vi "Test Copy To Raw Memory ARGB.vi"(8 "error in (no error)":errorcluster, 11 "Test Case In":refnum<class "01_Image.lvclass">) -> (0 "error out":errorcluster, 3 "Test Case Out":refnum<class "01_Image.lvclass">)   [LabVIEW 2020, in "test.lvlib" / "01_Image.lvclass"]
uses:
  01_Image.lvclass
  C:/Program Files (x86)/National Instruments/LabVIEW 2026/vi.lib/Astemes/LUnit/Test Case.lvclass
  common/Image Size (Integer).ctl
  image/Raw Memory Information.ctl
  image/Raw Memory Information Dimension.ctl
  <vilib>/Astemes/LUnit/Test Case.lvclass/Test Case.ctl
  4993e8ee-a06a-463a-9684-69129f64d5ce.vi
  image/New Image.vi
  image/New Image (ARGB Preallocated).vi
  image/Copy Array to Image.vi
  image/Copy Array to Image (ARGB).vi
  image/Copy Image to Memory Address (ARGB).vi/01eda17f-9221-4e43-bf47-cf9d986167a3.vi
  <vilib>/Astemes/LUnit/Core/LUnit Test Case/Private/Append Pass Result.vi
  <vilib>/Astemes/LUnit/Core/LUnit Test Case/Private/Append Fail Result.vi
  4993e8ee-a06a-463a-9684-69129f64d5ce.vi/9c5d11cd-9439-4240-a1ee-d9baace9c924.vi
  image/New Image (ARGB Preallocated).vi/3321fa97-f432-4e1e-8db9-a0df79aed21b.vi
  image/ARGB Colour to U32 Pixel Value.vi
  <vilib>/Astemes/LUnit/Core/LUnit Test Case/Private/Run In UI.vi
  <vilib>/Utility/error.llb/Clear Errors.vi
  <vilib>/Utility/error.llb/Error Cluster From Error Code.vi
  <vilib>/picture/pixmap.llb/Flatten Pixmap.vi
  image/image.lvlib
  common/common.lvlib
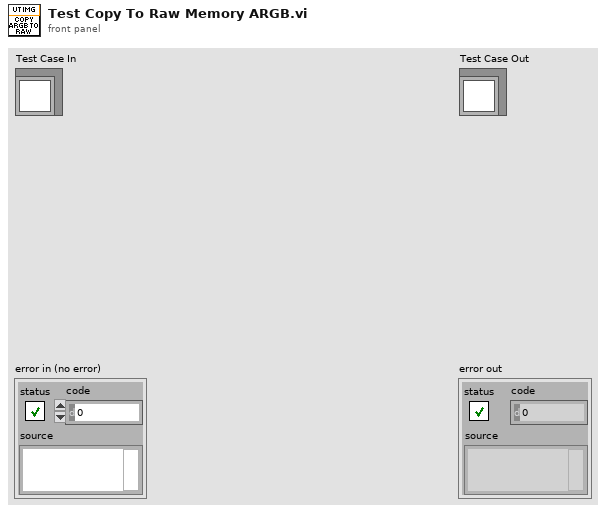
[diagram p1: front panel]
types:
  T1 = typedef "common.lvlib/Image Size (Integer).ctl" = cluster{"Width":u16, "Height":u16}
  T2 = typedef "image.lvlib/ARGB Image.ctl" = refnum<data-value>
  T3 = typedef "image.lvlib/Raw Memory Information.ctl" = cluster{"Memory Address":u64, "Dimension 0":T4, "Dimension 1":T4}
  T4 = typedef "image.lvlib/Raw Memory Information Dimension.ctl" = cluster{"Size":u16, "Stride":i32}
  T5 = cluster{"pointer":u64, "size_0":u32, "stride_0":i32, "size_1":u32, "stride_1":i32, "element size":u32, "subarray?":bool}
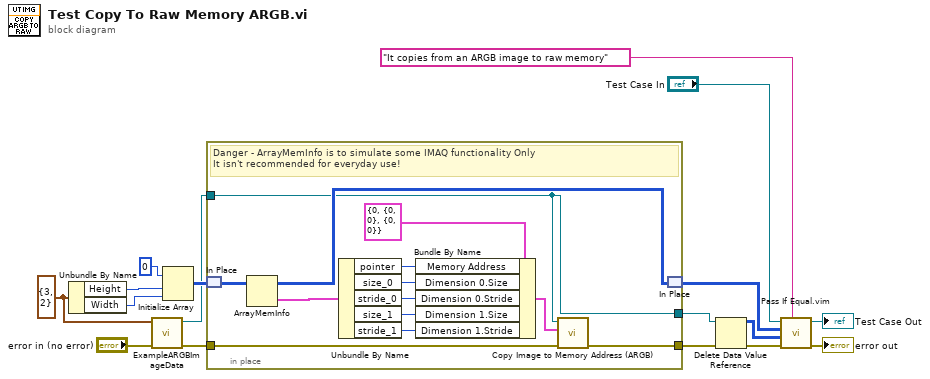
[diagram p0: block diagram]
diagram:
  w13 = T1 {"Width"=3, "Height"=2} ("Image Size")
  n1 = Unbundle By Name(w13) -> ("Height"=w12:u16, "Width"=w11:u16)
  n2 = call "ExampleARGBImageData.vi"("error in (no error)"="error in (no error)", "Image Size"=w13) -> ("error out"=w6:errorcluster, "Data Value Reference out"=w5:T2)  [unwired: 6 in, 2 out]
  n3 = Initialize Array(u32 0, w12, w11) -> (w9:u32[][])
  n4 = in-place "In Place Element Structure" {
    in-place-border: w6 -> [w19]
    in-place-border: [w22] -> w10
    in-place-border: w5 -> [w18]
    in-place-border: [w18] -> w3
    # "Danger - ArrayMemInfo is to simulate some IMAQ functionality Only\nIt isn't recommended for everyday use!"
    n5 = in-place-match #1(w9) -> (w20:u32[][])
    n6 = ArrayMemInfo(3:w20) -> (0:w30:T5, 1:w21:u32[][])
    n7 = Unbundle By Name(w30) -> ("pointer"=w28:u64, "size_0"=w26:u32, "stride_0"=w25:i32, "size_1"=w23:u32, "stride_1"=w24:i32)
    n8 = Bundle By Name(cluster=T3 {"Memory Address"=0, "Dimension 0"={"Size"=0, "Stride"=0}, "Dimension 1"={"Size"=0, "Stride"=0}} ("Destination"), "Memory Address"=w28, "Dimension 0.Size"=w26, "Dimension 0.Stride"=w25, "Dimension 1.Size"=w23, "Dimension 1.Stride"=w24) -> (w27:T3)
    n9 = call "Copy Image to Memory Address (ARGB).vi"("error in (no error)"=w19, "Destination"=w27, "ARGB Image Source in"=w18) -> ("error out"=w22:errorcluster)  [unwired: 7 in, 1 out]
    n10 = in-place-match #1(w21) -> (w2:u32[][])
  }
  n11 = Delete Data Value Reference(data value reference=w3, error in=w10) -> (data value=w1:u32[][], error out=w4:errorcluster)
  n12 = call "Pass If Equal.vim"("Description"="It copies from an ARGB image to raw memory", "error in (no error)"=w4, "Actual"=w1, "Expected"=w2, "LUnit Test Case In"="Test Case In") -> ("error out"=→"error out":errorcluster, "LUnit Test Case Out"=→"Test Case Out":refnum<class "01_Image.lvclass">)  [unwired: 5 in]
